vi "ContRunAux.vi"(4 "ControllerSettingsRef":refnum<vi>, 6 "CtrlRefsin":T3, 7 "Aux chart ref in":refnum<vi>, 8 "error in (no error)":errorcluster, 10 "Aux pulse in":T4, 11 "Main Pulse In":T4) -> (0 "error out":errorcluster, 2 "Aux stopped":bool, 3 "Main Pulse Out":T4)   [LabVIEW 2019]
uses:
  PulseControl.ctl
  Compiler/Params.ctl
  controls/xAOMSettings/XAOMsetting.xctl
  controls/PowerStableSettings.ctl
  controls/FluoSettings.ctl
  controls/ControllerSettings.ctl
  controls/CompCoilControl.ctl
  controls/GlobalExp.vi
  Global.lvlib
panel:
  in  "Cluster":T1
  in  "FluoCtrl":T2
  in  "image size":cluster{"xpixels":i32, "ypixels":i32}
  # "Current lock :"
  # "Unlock if :"
  # "Probability lock :"
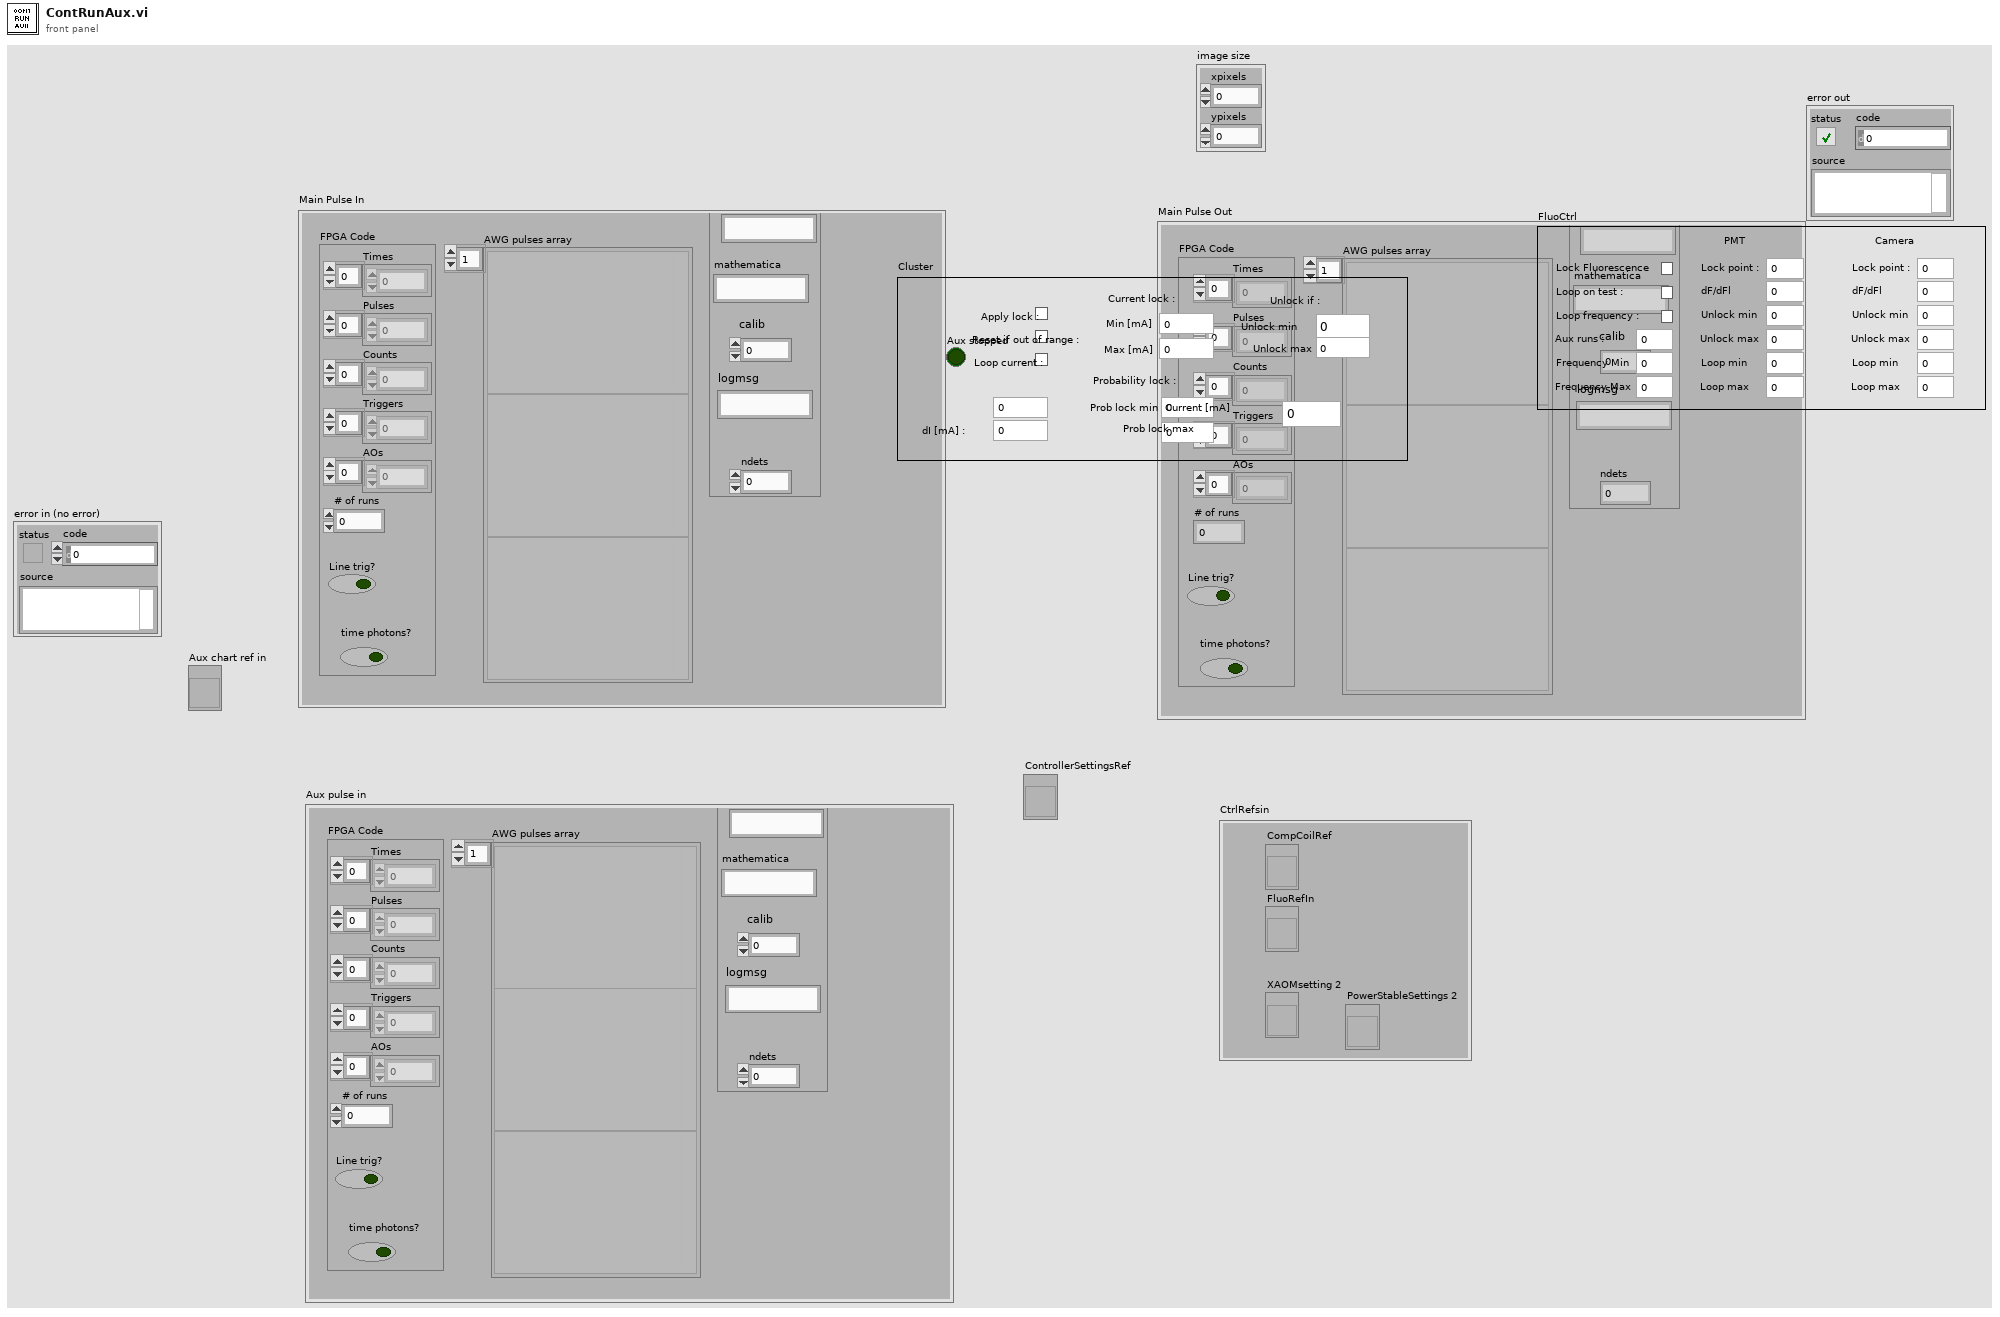
[diagram p1: front panel]
types:
  T1 = typedef "CompCoilControl.ctl" = cluster{"Min [mA]":dbl, "Max [mA]":dbl, "Apply lock :":bool, "Unlock min":dbl, "Unlock max":dbl, "Loop current :":bool, "Reset if out of range :":bool, "Aux runs :":i32, "dI [mA] :":dbl, "Prob lock min ":dbl, "Prob lock max":dbl, "Current [mA]":dbl}
  T2 = typedef "FluoSettings.ctl" = cluster{"Lock Fluorescence":bool, "Aux runs : ":i32, "Loop on test :":bool, "Loop frequency : ":bool, "Frequency Min":dbl, "Frequency Max":dbl, "PMT":cluster{"Lock point : ":dbl, "dF/dFl":dbl, "Unlock min":dbl, "Unlock max":dbl, "Loop min":dbl, "Loop max":dbl}, "Camera":cluster{"Lock point : ":dbl, "dF/dFl":dbl, "Unlock min":dbl, "Unlock max":dbl, "Loop min":dbl, "Loop max":dbl}}
  T3 = cluster{"CompCoilRef":refnum<vi>, "FluoRefIn":refnum<vi>, "XAOMsetting 2":refnum<vi>, "PowerStableSettings 2":refnum<vi>}
  T4 = typedef "PulseControl.ctl" = cluster{"FPGA Code":cluster{"Times":u32[], "Pulses":u64[], "Counts":u8[], "Triggers":u8[], "AOs":u8[], "# of runs":i32, "Line trig?":bool, "time photons?":bool}, "AWG pulses array":variant[], "Params":T5}
  T5 = typedef "Params.ctl" = cluster{"steps":i16, "runs":i16, "comment":string, "mathematica":string, "calib":i8, "logmsg":string, "ndets":i16}
  T6 = typedef "MasterExpControl.ctl" = cluster{"Main Steps":dbl, "Main Runs":dbl, "ExpStatus":enum16{"Innit", "Stop", "Idle", "MainRunning", "AuxRunning"}, "Main Current Step":dbl, "ExpNum":dbl, "NewData":bool, "date":string, "command":string, "Stop":bool, "Pause":bool, "Mathematica":string, "Main/Meta":bool, "UpdateMath":bool, "Camera":bool, "MetaExpOver":bool, "NextMetaExp":bool}
  T7 = enum16{"Innit", "Stop", "Idle", "MainRunning", "AuxRunning"}
  T8 = cluster{"Lock outside range?":bool, "Kill lock?":bool, "Is probe in lock range?":bool, "Probe lock successful?":bool}
  T9 = cluster{"readout":u32[][], "kinetic series data":i32[][][][], "camera dim":cluster{i32, i32, i32, i32}}
  T10 = cluster{"Lock outside range?":bool, "Kill lock?":bool, "Is fluor in lock range?":bool, "Fluor lock successful?":bool}
  T11 = cluster{"HighPowerNum":dbl, "LowPowerNum":dbl, "PIDnum":dbl, "DeltaFreq":dbl, "BaseFreq":dbl, "AOMout":dbl, "ButtonSelected":enum16{"PID", "Low", "High"}, "AO3":bool}
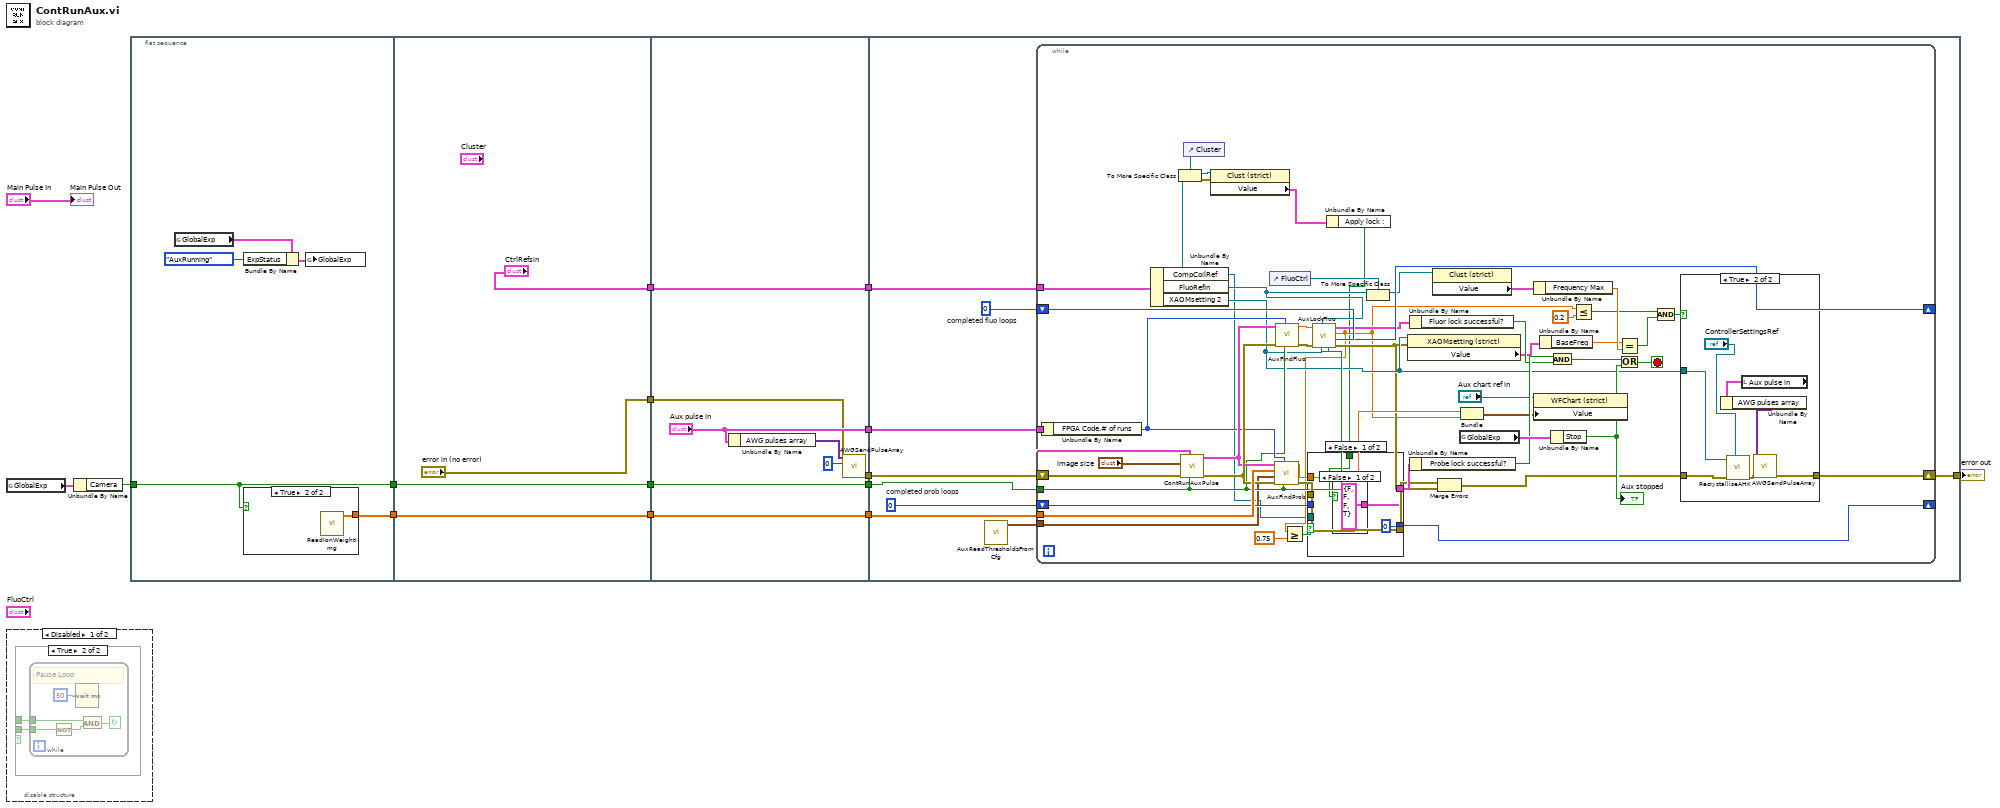
[diagram p0: block diagram]
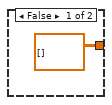
[diagram p2: hidden frame]
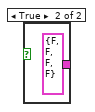
[diagram p3: hidden frame]
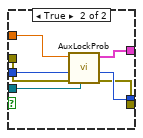
[diagram p4: hidden frame]
diagram:
  n1 = global read "GlobalExp.vi" "GlobalExp"() -> (w13:T6)
  n2 = disable-structure shown="Disabled" {
    frame Disabled {
      n3 = case shown="True" {
        selector: _ -> [_ _]
        tunnel: _ -> [_ w17]
        tunnel: _ -> [_ w16]
        frame False {
        }
        frame True {
          n4 = while {
            tunnel: w17 -> [w20]
            tunnel: w16 -> [w18]
            stop <- w21 continue-if-true
            # "Pause Loop"
            n5 = Not(x=w18) -> (.not. x?=w19:bool)
            n6 = Wait (ms)(milliseconds to wait=u32 50) -> ()  [unwired: 1 out]
            n7 = And(x=w20, y=w19) -> (x .and. y?=w21:bool)
          }
        }
      }
    }
    frame Enabled {
    }
  }
  n8 = Unbundle By Name(w13) -> ("Camera"=w12:bool)
  n9 = flat-sequence {
    tunnel: w12 -> [w23]
    tunnel: [w24] -> w7
    tunnel: [w23] -> w5
    tunnel: w7 -> [w33]
    tunnel: [w33] -> w6
    tunnel: w5 -> [w32]
    tunnel: [w32] -> w4
    tunnel: ["CtrlRefsin"] -> w2
    tunnel: ["error in (no error)"] -> w1
    tunnel: w6 -> [w41]
    tunnel: [w41] -> w11
    tunnel: w4 -> [w40]
    tunnel: [w40] -> w10
    tunnel: ["Aux pulse in"] -> w9
    tunnel: [w36] -> w8
    tunnel: [w35] -> w3
    tunnel: w2 -> [w35]
    tunnel: w1 -> [w34]
    tunnel: w11 -> [w50]
    tunnel: [w47] -> w14
    tunnel: w10 -> [w46]
    tunnel: w9 -> [w45]
    tunnel: w8 -> [w42]
    tunnel: w3 -> [w43]
    frame #0 {
      n10 = global read "GlobalExp.vi" "GlobalExp"() -> (w25:T6)
      n11 = Bundle By Name(cluster=w25, "ExpStatus"=T7."AuxRunning") -> (w26:T6)
      n12 = case shown="True" w23 {
        tunnel: [dbl[][] [] ("ion weight") w29] -> w24
        frame False {
        }
        frame True {
          n13 = call "ReadIonWeightImg.vi"() -> ("ion weight"=w29:dbl[][])  [unwired: 11 in]
        }
      }
      n14 = global write "GlobalExp.vi" "GlobalExp"(w26) -> ()
    }
    frame #1 {
    }
    frame #2 {
      n15 = Unbundle By Name("Aux pulse in") -> ("AWG pulses array"=w39:variant[])
      n16 = call "AWGSendPulseArray.vi"("error in (no error)"=w34, "Step Number"=0, "AWG pulses array"=w39) -> ("error out"=w36:errorcluster)  [unwired: 8 in]
    }
    frame #3 {
      w48 = 0  # completed fluo loops
      w49 = 0  # completed prob loops
      n17 = call "AuxReadThresholdsFromCfg.vi"() -> ("threshholds"=w44:cluster{"t1 pmt":i32, "t1 camera":i32})  [unwired: 11 in]
      n18 = while {
        tunnel: w46 -> [w91]
        tunnel: w50 -> [w101]
        shift-right: [w95] -> _
        shift-left: w49 -> [w96]
        shift-right: [w92] -> _
        shift-left: w48 -> [w93]
        shift-right: [w73] -> w47
        shift-left: w42 -> [w102]
        tunnel: w45 -> [w78]
        tunnel: w44 -> [w77]
        tunnel: w43 -> [w57]
        stop <- w85 stop-if-true
        n19 = Unbundle By Name(w78) -> ("FPGA Code.# of runs"=w98:i32)
        n20 = Unbundle By Name(w57) -> ("CompCoilRef"=w52:refnum<vi>, "FluoRefIn"=w68:refnum<vi>, "XAOMsetting 2"=w72:refnum<vi>)
        n21 = call "ContRunAuxPulse.vi"("camera"=w91, "Aux pulse in"=w78, "error in (no error)"=w102, "image size"="image size") -> ("error out"=w100:errorcluster, "READOUT"=w99:T9)  [unwired: 6 in]
        n22 = control-ref of="Cluster"() -> (w55:refnum<vi>)
        n23 = To More Specific Class(target class=w55, reference=w52) -> (specific class reference=w56:refnum<vi>, error out=w54:errorcluster)  [unwired: 1 in]
        n24 = property class="Clust (strict)"(reference=w56, error in=w54) -> ("Value"=w53:T1)  [unwired: 2 out]
        n25 = control-ref of="FluoCtrl"() -> (w69:refnum<vi>)
        n26 = call "AuxFindProb.vi"("camera?"=w91, "nruns"=w98, "error in"=w100, "threshholds"=w77, "camera weight img"=w101, "READOUT"=w99) -> ("error out"=w97:errorcluster, "prob"=w83:dbl)  [unwired: 4 in]
        n27 = call "AuxFindFluo.vi"("camera?"=w91, "nruns"=w98, "error in (no error)"=w100, "READOUT"=w99) -> ("error out"=w94:errorcluster, "av fluo"=w82:dbl)  [unwired: 6 in]
        n28 = call "AuxLockFluo.vi"("XAOMsetting 2"=w72, "Camera?"=w91, "FluoRefIn"=w68, "error in"=w94, "Completed loops in"=w93, "fluo in"=w82) -> ("error out"=w71:errorcluster, "Completed loops out"=w92:u32, "fluo normalized"=w59:dbl, "fl lock bools"=w89:T10)  [unwired: 2 in]
        n29 = Greater Or Equal?(x=w59, y=0.75) -> (x >= y?=w60:bool)
        n30 = Unbundle By Name(w53) -> ("Apply lock :"=w51:bool)
        n31 = case shown="False" w60 {
          tunnel: w97 -> [w107 w116]
          tunnel: w96 -> [_ w115]
          tunnel: [u32 0 ("Completed loops out") w114] -> w95
          tunnel: [w106 w113] -> w90
          tunnel: w83 -> [_ w112]
          tunnel: [w107 w111] -> w79
          tunnel: w52 -> [_ w110]
          tunnel: w51 -> [w104 _]
          frame False {
            n32 = case shown="False" w104 {
              tunnel: [T8 {"Lock outside range?"=FALSE, "Kill lock?"=FALSE, "Is probe in lock range?"=FALSE, "Probe lock successful?"=TRUE} ("probe lock bools") T8 {"Lock outside range?"=FALSE, "Kill lock?"=FALSE, "Is probe in lock range?"=FALSE, "Probe lock successful?"=FALSE} ("probe lock bools")] -> w106
              frame False {
              }
              frame True {
              }
            }
          }
          frame True {
            n33 = call "AuxLockProb.vi"("CompCoilRef"=w110, "error in"=w116, "Completed loops in"=w115, "prob in"=w112) -> ("error out"=w111:errorcluster, "Completed loops out"=w114:u32, "probe lock bools"=w113:T8)  [unwired: 5 in]
          }
        }
        n34 = To More Specific Class(target class=w69, reference=w68) -> (specific class reference=w67:refnum<vi>)  [unwired: 1 in, 1 out]
        n35 = property class="XAOMsetting (strict)"(reference=w72, error in=w71) -> ("Value"=w70:T11)  [unwired: 2 out]
        n36 = Unbundle By Name(w90) -> ("Probe lock successful?"=w88:bool)
        n37 = Unbundle By Name(w89) -> ("Fluor lock successful?"=w87:bool)
        n38 = property class="Clust (strict)"(reference=w67) -> ("Value"=w66:T2)  [unwired: 1 in, 2 out]
        n39 = Merge Errors(w79, w71) -> (w74:errorcluster)
        n40 = global read "GlobalExp.vi" "GlobalExp"() -> (w103:T6)
        n41 = Bundle("prob"=w83, "fluo normalized"=w59) -> (w80:cluster{"prob":dbl, "fluo normalized":dbl})  [unwired: 1 in]
        n42 = Unbundle By Name(w66) -> ("Frequency Max"=w65:dbl)
        n43 = property class="WFChart (strict)"(reference="Aux chart ref in", "Value"=w80) -> ()  [unwired: 1 in, 2 out]
        n44 = Unbundle By Name(w70) -> ("BaseFreq"=w64:dbl)
        n45 = And(x=w88, y=w87) -> (x .and. y?=w86:bool)
        n46 = Unbundle By Name(w103) -> ("Stop"=w76:bool)
        "Aux stopped" <- w76
        n47 = Less Or Equal?(x=w59, y=0.2) -> (x <= y?=w62:bool)
        n48 = Equal?(x=w64, y=w65) -> (x = y?=w61:bool)
        n49 = Or(x=w86, y=w76) -> (x .or. y?=w85:bool)
        n50 = And(x=w62, y=w61) -> (x .and. y?=w63:bool)
        n51 = case shown="True" w63 {
          tunnel: w74 -> [w117 w124]
          tunnel: w72 -> [_ w123]
          tunnel: [w117 w121] -> w73
          frame False {
          }
          frame True {
            n52 = call "RecrystalliseAHK.vi"("ControllerSettingsRef"="ControllerSettingsRef", "error in (no error)"=w124, "XAOMsetting"=w123) -> ("error out"=w122:errorcluster)  [unwired: 8 in]
            n53 = local read "Aux pulse in"() -> (w120:T4)
            n54 = Unbundle By Name(w120) -> ("AWG pulses array"=w119:variant[])
            n55 = call "AWGSendPulseArray.vi"("error in (no error)"=w122, "AWG pulses array"=w119) -> ("error out"=w121:errorcluster)  [unwired: 9 in]
          }
        }
      }
    }
  }
  "error out" <- w14
  "Main Pulse Out" <- "Main Pulse In"
